vi "Set camera sensor mode.vi"(7 "Error In":errorcluster, 9 "mode":i32(ring)=27 items=["BGRA8Packed"=0, "BGR8Packed"=1, "BGR565Packed"=2, "BGR5Packed"=3, "Mono8"=6, "SensorRaw8"=11, "UYVYPacked"=12, "UYVYMonoPacked"=13, "UYVYBayerPacked"=14, "CBYCRYPacked"=23, "BGRY8Packed"=24, "BGR10Packed"=25, "Mono12"=26, "SensorRaw12"=27, "Mono16"=28, "SensorRaw16"=29, "BGR12Unpacked"=30, "BGRA12Unpacked"=31, "Jpeg"=32, "BGR10Unpacked"=35, "RGBA8Packed"=128, "RGB8Packed"=129, "RGBY8Packed"=152, "RGB10Packed"=153, "RGB12Unpacked"=158, "RGBA12Unpacked"=159, "RGB10Unpacked"=163, "RGB8Planar"=8321, "PreferPackedSourceFormat"=16384], 10 "Camera reference in":refnum<k24>) -> (0 "Error Out":errorcluster, 3 "Camera reference out":refnum<k24>)   [LabVIEW 2017]
uses:
  C:/Program Files/National Instruments/LabVIEW 2017/instr.lib/IDS/ueye.NET/uEyeDotNet.dll
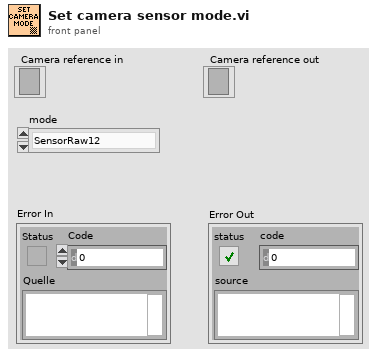
[diagram p1: front panel]
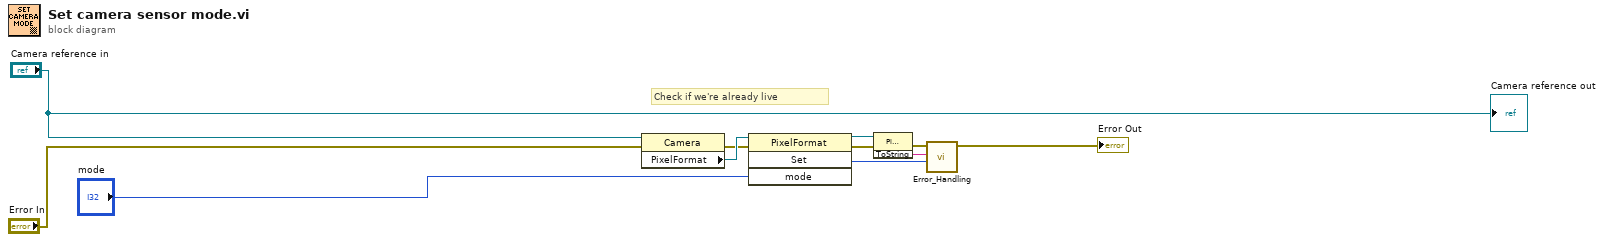
[diagram p0: block diagram]
diagram:
  # "Check if we're already live"
  n1 = property class="Camera"(reference="Camera reference in", error in="Error In") -> (error out=w5:errorcluster, "PixelFormat"=w6:refnum<k24>)  [unwired: 1 out]
  n2 = invoke class="PixelFormat" method="Set"(reference=w6, error in=w5, "mode"="mode") -> (reference out=w9:refnum<k24>, error out=w10:errorcluster, "Set"=w11:i32)  [unwired: 1 in, 1 out]
  n3 = invoke class="PixelFormat" method="ToString"(reference=w9, error in=w10) -> (error out=w7:errorcluster, "ToString"=w8:string)  [unwired: 1 in, 1 out]
  n4 = call <instrlib>:"Error_Handling.vi"("Error Code"=w11, "Error String"=w8, "Error In"=w7) -> ("Error Out"=→"Error Out":errorcluster)  [unwired: 8 in]
  "Camera reference out" <- "Camera reference in"
